vi "Set Power.vi"(8 "error in (no error)":errorcluster, 10 "Power":dbl, 11 "Lauda Settings In":T1) -> (0 "error out":errorcluster, 1 "Connection Error":bool, 3 "Lauda Settings Out":T1)   [LabVIEW 2021, in "Lauda TCU.lvlib"]
uses:
  Lauda TCU.lvlib
  Lauda Settings.ctl
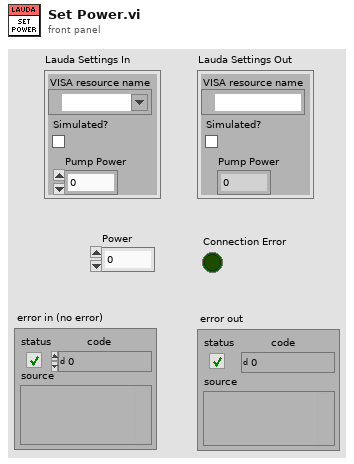
[diagram p1: front panel]
types:
  T1 = typedef "Lauda TCU.lvlib/Lauda Settings.ctl" = cluster{"VISA resource name":refnum<visa-resource-name>, "Simulated?":bool, "Pump Power":i32}
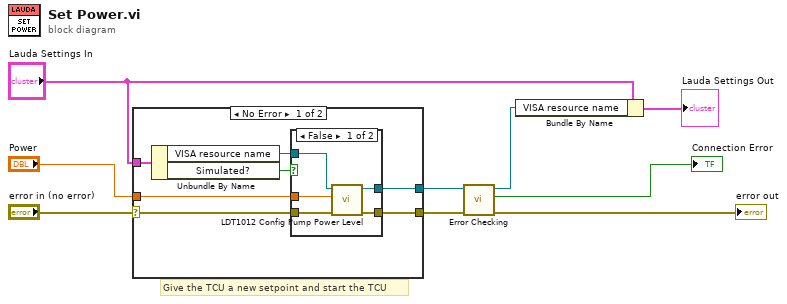
[diagram p0: block diagram]
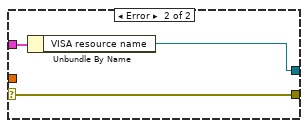
[diagram p3: hidden frame]
diagram:
  # "Give the TCU a new setpoint and start the TCU"
  n1 = case shown="No Error" "error in (no error)" {
    selector: "error in (no error)" -> [w16 w26]
    tunnel: "Lauda Settings In" -> [w12 w25]
    tunnel: [w15 w26] -> w7
    tunnel: [w14 w24] -> w8
    tunnel: "Power" -> [w10 _]
    frame No Error {
      n2 = Unbundle By Name(w12) -> ("VISA resource name"=w11:refnum<visa-resource-name>, "Simulated?"=w13:bool)
      n3 = case shown="False" w13 {
        tunnel: w16 -> [w19 w23]
        tunnel: [w18 w23] -> w15
        tunnel: [w17 w22] -> w14
        tunnel: w11 -> [w20 w22]
        tunnel: w10 -> [w21 _]
        frame False {
          n4 = call "LDT1012 Config Pump Power Level.vi"("error in (no error)"=w19, "Pump Power Level (2: Default)"=w21, "VISA session"=w20) -> ("error out"=w18:errorcluster, "dup VISA session"=w17:refnum<visa-resource-name>)  [unwired: 7 in]
        }
        frame True {
        }
      }
    }
    frame Error {
      n5 = Unbundle By Name(w25) -> ("VISA resource name"=w24:refnum<visa-resource-name>)
    }
  }
  n6 = call "Error Checking.vi"("error in (no error)"=w7, "VISA resource name"=w8) -> ("error out"=→"error out":errorcluster, "Connection Error"=→"Connection Error":bool, "VISA resource name"=w5:refnum<visa-resource-name>)  [unwired: 7 in]
  n7 = Bundle By Name(cluster="Lauda Settings In", "VISA resource name"=w5) -> (→"Lauda Settings Out":T1)
